vi "readFromXML.vi"(8 "error in (no error)":errorcluster, 10 "XML in":string, 11 "PointAdd in":refnum<class "PointAdd.lvclass">) -> (0 "error out":errorcluster, 3 "PointAdd out":refnum<class "PointAdd.lvclass">)   [LabVIEW 2022 SP3, in "TCSDataDefinitions.lvlib" / "TCSCommand.lvlib" / "PointingFileCommands.lvlib" / "PointAdd.lvclass"]
uses:
  PointAdd.lvclass
  PointingFileCommands/PointingFileCommands.lvclass
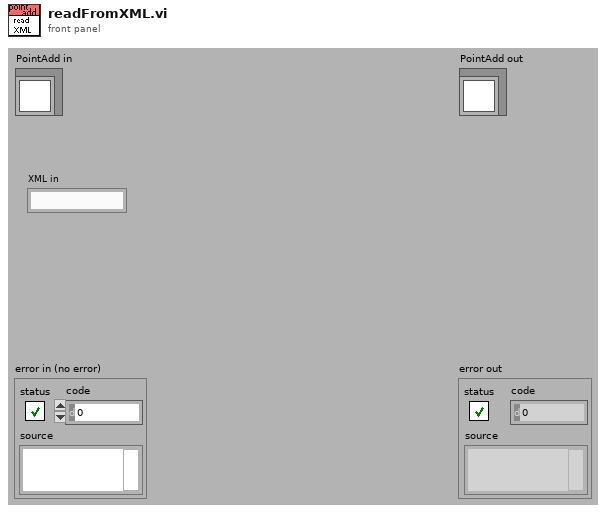
[diagram p1: front panel]
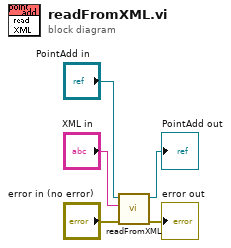
[diagram p0: block diagram]
diagram:
  n1 = call-parent "readFromXML.vi"("error in (no error)"="error in (no error)", "XML in"="XML in", "PointingFileCommands in"="PointAdd in") -> ("error out"=→"error out":errorcluster, "PointingFileCommands out"=→"PointAdd out":refnum<class "PointAdd.lvclass">)  [unwired: 7 out]
